vi "Save Batt Voltage.vi"(4 "Battery Capture 310":u64, 6 "Battery Capture 280":u64, 8 "error in (no error)":errorcluster, 11 "[A/Ds]":dbl[][](array[numeric])) -> (2 "Pass/Fail #":i32, 3 "Pass?":bool)   [LabVIEW 2013]
uses:
  InputScript states.ctl
  <vilib>/Utility/NIReport.llb/NI_report.lvclass
  <vilib>/addons/_office/excel.llb/Excel Easy Table (num).vi
  <vilib>/addons/_office/excel.llb/Excel Get Data ([str]).vi
  <vilib>/Utility/NIReport.llb/Excel/NI_Excel.lvclass
  <vilib>/addons/_office/NI_ReportGenerationToolkit.lvlib
panel:
  out "error out":errorcluster
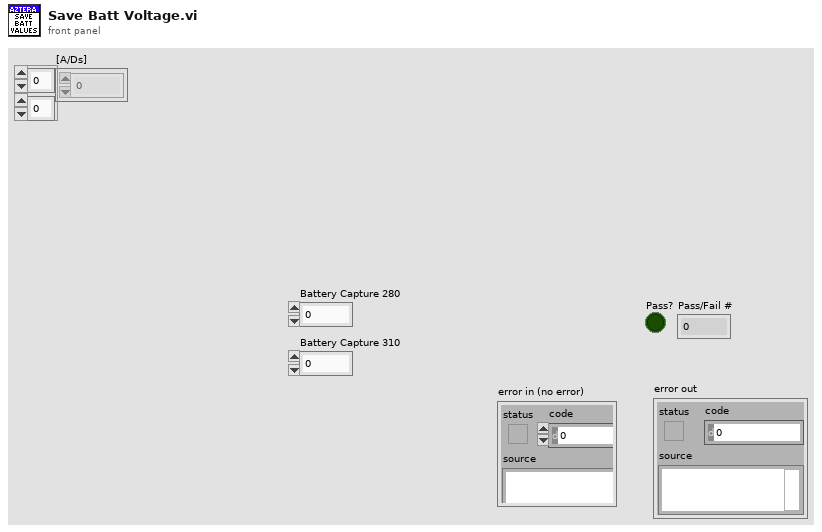
[diagram p1: front panel]
types:
  T1 = typedef "InputScript states.ctl" = enum16{"Open Template", "Write Values", "Read Results", "Close Template"}
  T2 = enum16{"maximized", "minimized", "normal", "no change"}
  T3 = enum16{"Standard Report", "HTML", "Word", "Excel"}
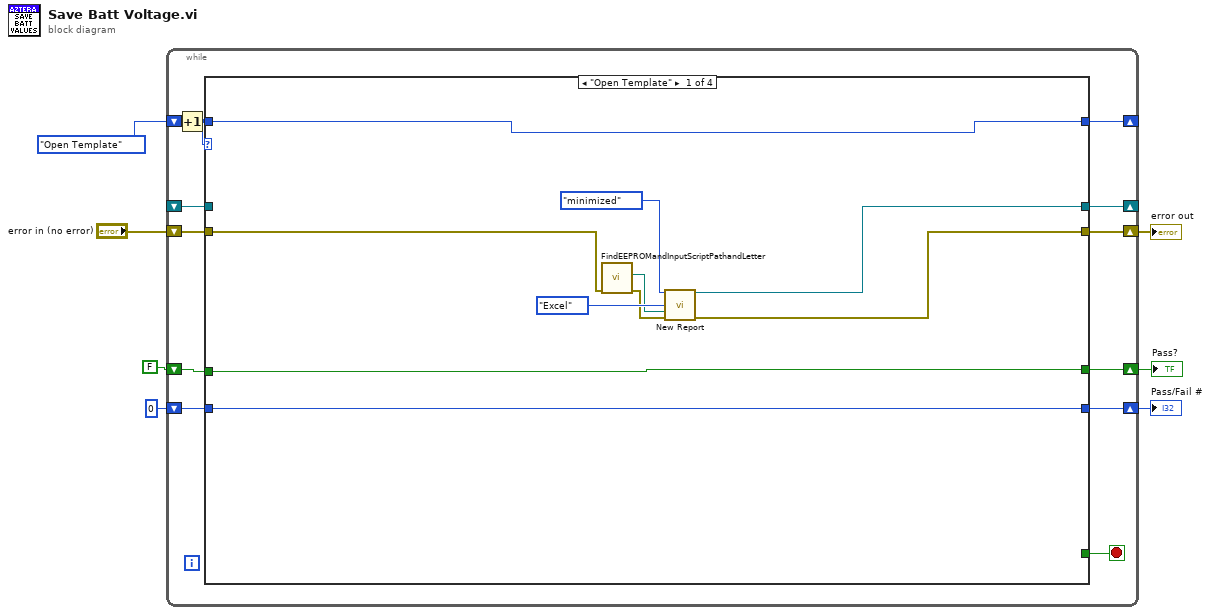
[diagram p0: block diagram]
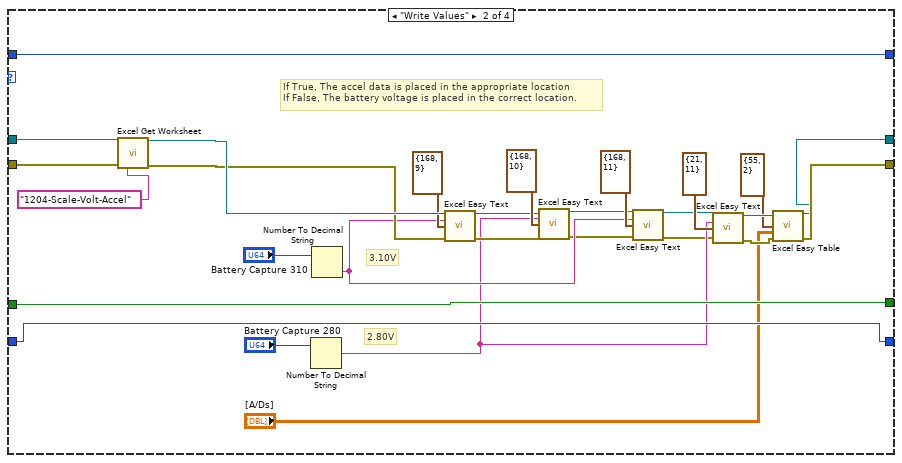
[diagram p2: hidden frame]
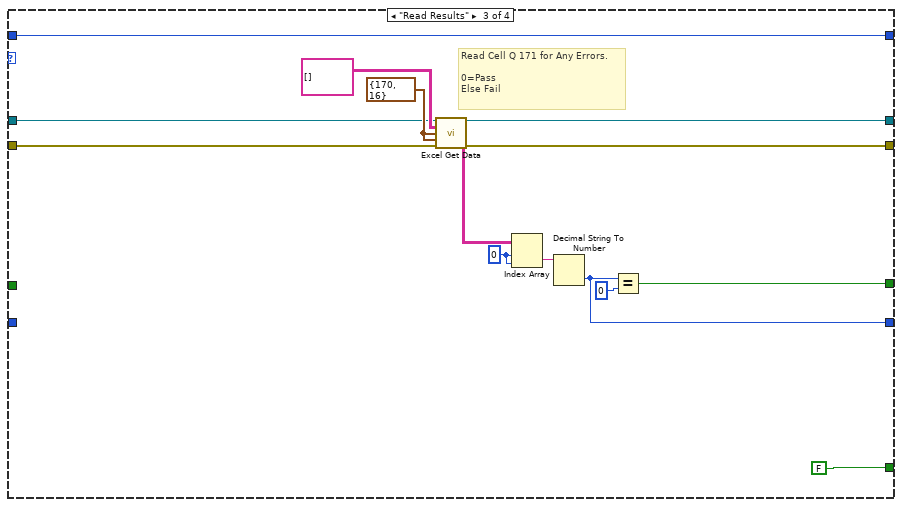
[diagram p3: hidden frame]
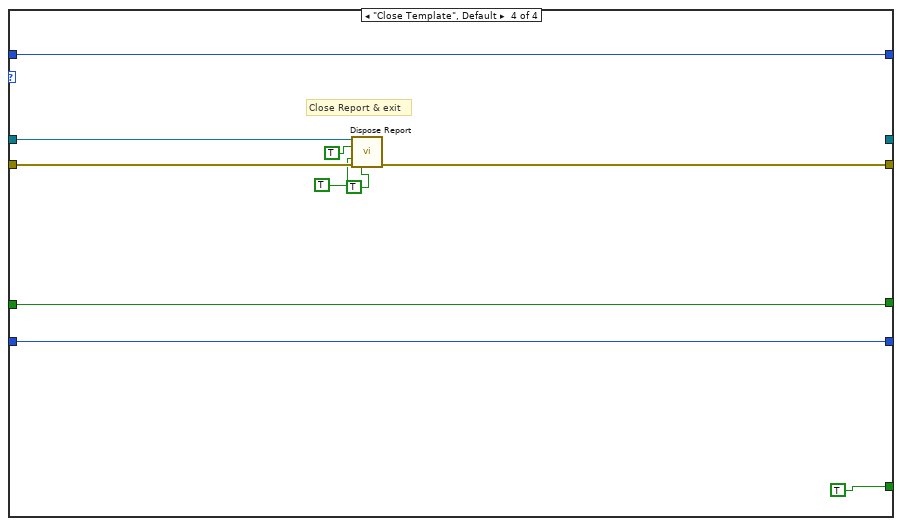
[diagram p4: hidden frame]
diagram:
  n1 = while {
    shift-right: [w18] -> _
    shift-left: _ -> [w17]
    shift-right: [w16] -> w1
    shift-left: "error in (no error)" -> [w15]
    shift-right: [w12] -> _
    shift-left: InputScript_states."Open Template" -> [w14]
    shift-right: [w11] -> w5
    shift-left: 0 -> [w9]
    shift-right: [w10] -> w4
    shift-left: FALSE -> [w8]
    stop <- w19 stop-if-true
    n2 = Increment(x=w14) -> (x+1=w13:T1)
    n3 = case shown="\"Open Template\"" w14 {
      tunnel: [_ _ FALSE TRUE] -> w19
      tunnel: [w29 w32 w66 _] -> w18
      tunnel: w17 -> [_ w56 w59 w80]
      tunnel: [w28 w34 w65 w78] -> w16
      tunnel: w15 -> [w21 w54 w58 w79]
      tunnel: w13 -> [w27 w57 w71 w76]
      tunnel: [w27 w57 w71 w76] -> w12
      tunnel: [w24 w51 w61 w74] -> w11
      tunnel: [w23 w50 w69 w73] -> w10
      tunnel: w9 -> [w24 w51 _ w74]
      tunnel: w8 -> [w23 w50 _ w73]
      frame "Open Template" {
        n4 = call "FindEEPROMandInputScriptPathandLetter.vi"("Error In"=w21) -> ("Error Out"=w20:errorcluster, "Engr Result Path"=w22:path)  [unwired: 6 in, 1 out]
        n5 = call <vilib>:"New Report.vi"("window state (normal)"=T2."minimized", "report type"=T3."Excel", "template (empty)"=w22, "error in (no error)"=w20) -> ("report out"=w29:refnum<class "NI_report.lvclass">, "error out"=w28:errorcluster)  [unwired: 10 in]
      }
      frame "Write Values" {
        # "3.10V"
        # "2.80V"
        # "If True, The accel data is placed in the appropriate location\nIf False, The battery voltage is placed in the correct location."
        n6 = call <vilib>:"Excel Get Worksheet.vi"("report in"=w56, "error in (no error)"=w54, "name (\"\")"="1204-Scale-Volt-Accel" ("name (\"\")")) -> ("report out"=w55:refnum<class "NI_report.lvclass">, "error out"=w53:errorcluster)  [unwired: 11 in]
        n7 = Number To Decimal String(number="Battery Capture 280") -> (decimal integer string=w38:string)  [unwired: 1 in]
        n8 = Number To Decimal String(number="Battery Capture 310") -> (decimal integer string=w42:string)  [unwired: 1 in]
        n9 = call <vilib>:"Excel Easy Text.vi"("report in"=w55, "text"=w42, "start (-1, -1)"=cluster{"row":i32, "column":i32} {"row"=168, "column"=9}, "error in (no error)"=w53) -> ("report out"=w47:refnum<class "NI_report.lvclass">, "error out"=w46:errorcluster)  [unwired: 7 in, 3 out]
        n10 = call <vilib>:"Excel Easy Text.vi"("report in"=w47, "text"=w38, "start (-1, -1)"=cluster{"row":i32, "column":i32} {"row"=168, "column"=10}, "error in (no error)"=w46) -> ("report out"=w41:refnum<class "NI_report.lvclass">, "error out"=w40:errorcluster)  [unwired: 7 in, 3 out]
        n11 = call <vilib>:"Excel Easy Text.vi"("report in"=w41, "text"=w42, "start (-1, -1)"=cluster{"row":i32, "column":i32} {"row"=168, "column"=11}, "error in (no error)"=w40) -> ("report out"=w36:refnum<class "NI_report.lvclass">, "error out"=w37:errorcluster)  [unwired: 7 in, 3 out]
        n12 = call <vilib>:"Excel Easy Text.vi"("report in"=w36, "text"=w38, "start (-1, -1)"=cluster{"row":i32, "column":i32} {"row"=21, "column"=11}, "error in (no error)"=w37) -> ("report out"=w33:refnum<class "NI_report.lvclass">, "error out"=w35:errorcluster)  [unwired: 7 in, 3 out]
        n13 = call-poly <vilib>:"Excel Easy Table.vi"("report in"=w33, "start (0, 0)"=cluster{"row":i32, "column":i32} {"row"=55, "column"=2}, "text data"="[A/Ds]", "error in (no error)"=w35) -> ("report out"=w32:refnum<class "NI_report.lvclass">, "error out"=w34:errorcluster)  [unwired: 7 in, 3 out]
      }
      frame "Read Results" {
        w67 = cluster{"row":i32, "column":i32} {"row"=170, "column"=16} ("start (-1, -1)")
        w63 = 0
        # "Read Cell Q 171 for Any Errors. \n\n0=Pass\nElse Fail"
        n14 = call-poly <vilib>:"Excel Get Data.vi"("report in"=w59, "data type"=string[][] [], "start (-1, -1)"=w67, "end (-1, -1)"=w67, "error in (no error)"=w58) -> ("report out"=w66:refnum<class "NI_report.lvclass">, "data"=w64:string[][], "error out"=w65:errorcluster)  [unwired: 8 in]
        n15 = Index Array(array=w64, index (row)=w63, index (col)=w63) -> (element=w62:string)
        n16 = Decimal String To Number(string=w62) -> (number=w61:i32)  [unwired: 2 in, 1 out]
        n17 = Equal?(x=w61, y=0) -> (x = y?=w69:bool)
      }
      frame "Close Template", Default {
        # "Close Report & exit"
        n18 = call-dynamic "Dispose Report.vi"("report in"=w80, "wait until printing completed? (T)"=TRUE, "save changes? (F)"=TRUE, "error in (no error)"=w79, "close report? (T)"=TRUE) -> ("error out"=w78:errorcluster)  [unwired: 10 in]
      }
    }
  }
  "Pass/Fail #" <- w5
  "Pass?" <- w4
  "error out" <- w1
